vi "Full List.vi"(4 "Error in":errorcluster, 7 "Start Path\n(empty - Prompt)":path) -> (0 "Error out":errorcluster, 1 "Folders":path[](array[path]), 2 "# of files":i32, 3 "Files":path[](array[path]))   [LabVIEW 2011]
doc: "This VI searches for all the VIs in the hierarchy of a given VI and returns an array of their paths. \nEach VI is returned once in the list, regardless of how may times it appears in the hierarchy."
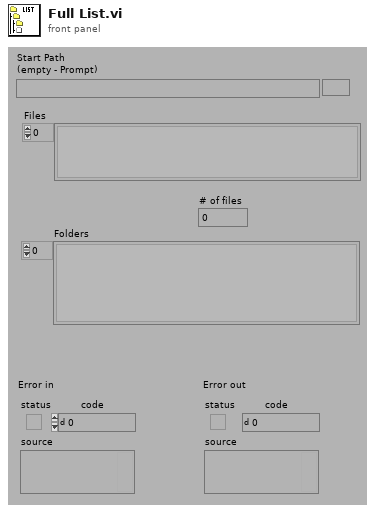
[diagram p1: front panel]
types:
  T1 = enum32{"existing file", "new file", "new or existing file", "existing dir", "new dir", "new or existing dir", "existing file (use LLBs)", "new file (use LLBs)", "new or existing file (use LLBs)", "new or existing file or directory (use LLBs)"}
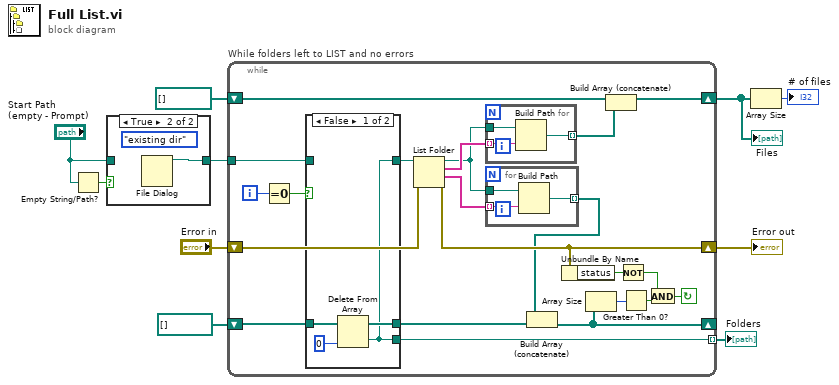
[diagram p0: block diagram]
diagram:
  n1 = Empty String/Path?(string/path="Start Path\n(empty - Prompt)") -> (empty?=w7:bool)
  n2 = case shown="True" w7 {
    tunnel: "Start Path\n(empty - Prompt)" -> [w11 _]
    tunnel: [w11 w12] -> w5
    frame False {
    }
    frame True {
      (unwired) T1."existing dir" ("select mode (2)")
      n3 = File Dialog() -> (3:w12:path)  [unwired: 1 in, 9 out]
    }
  }
  n4 = while "While folders left to LIST and no errors" {
    tunnel: w5 -> [w27]
    shift-left: path[] [] -> [w25]
    shift-right: [w22] -> _
    shift-left: path[] [] -> [w33]
    shift-right: [w32] -> w9
    shift-left: "Error in" -> [w34]
    shift-right: [w19] -> w3
    tunnel: [w13] -> w1 mode=indexing
    i -> [w29]
    stop <- w23 continue-if-true
    n5 = Equal To 0?(x=w29) -> (x = 0?=w28:bool)
    n6 = case shown="False" w28 {
      tunnel: [w38 w42] -> w26
      tunnel: w27 -> [_ w42]
      tunnel: w25 -> [w41 w43]
      tunnel: [w40 w43] -> w24
      tunnel: [w38 w42] -> w13
      frame False {
        n7 = Delete From Array(array=w41, index=0 ("Index")) -> (deleted portion=w38:path, array with subset deleted=w40:path[])  [unwired: 1 in]
      }
      frame True {
      }
    }
    n8 = List Folder(path=w26, error in=w34) -> (path out=w16:path, filenames=w31:string[], folder names=w15:string[], error out=w19:errorcluster)  [unwired: 2 out]
    n9 = for {
      tunnel: w31 -> [w46] mode=indexing
      tunnel: w16 -> [w45]
      tunnel: [w44] -> w30 mode=indexing
      n10 = Build Path(base path=w45, name or relative path=w46) -> (appended path=w44:path)
    }
    n11 = for {
      tunnel: w16 -> [w37]
      tunnel: w15 -> [w36] mode=indexing
      tunnel: [w35] -> w14 mode=indexing
      n12 = Build Path(base path=w37, name or relative path=w36) -> (appended path=w35:path)
    }
    n13 = Build Array (concatenate)(w14, w24) -> (w22:path[])
    n14 = Unbundle By Name(w19) -> ("status"=w18:bool)
    n15 = Array Size(array=w22) -> (size(s)=w21:i32)
    n16 = Build Array (concatenate)(w33, w30) -> (w32:path[])
    n17 = Not(x=w18) -> (.not. x?=w17:bool)
    n18 = Greater Than 0?(x=w21) -> (x > 0?=w20:bool)
    n19 = And(x=w17, y=w20) -> (x .and. y?=w23:bool)
  }
  "Error out" <- w3
  "Files" <- w9
  "Folders" <- w1
  n20 = Array Size(array=w9) -> (size(s)=→"# of files":i32)
